vi "ExecuteXML.vi"(0 "reference in":refnum<class "ViPER.lvclass">, 1 "XML_In":string, 3 "get_prototype":bool, 5 "error in (no error)":errorcluster) -> (14 "reference out":refnum<class "ViPER.lvclass">, 15 "XML_Out":string, 19 "error out":errorcluster)   [LabVIEW 2019]
doc: "### BSD License (http://www.opensource.org/licenses/bsd-license.php) Begin ###\n\nCopyright (c) 2018 Kurt Friday www.medulla.net\n\nAll rights reserved.\n\nRedistribution and use in source and binary forms, with or without\nmodification, are permitted provided that the following conditions are met:\n\n * Redistributions of source code must retain the above copyright\n notice, this list of conditions and the following disclaimer.\n\n * Redistributions in binary form must reproduce the above copyright\n notice, this list of conditions and the following disclaimer in the\n documentation and/or other materials provided with the distribution.\n\n * Neither the name of the <organization> nor the\n names of its contributors may be used to endorse or promote products\n derived from this software without specific prior written permission.\n\nTHIS SOFTWARE IS PROVIDED BY THE COPYRIGHT HOLDERS AND CONTRIBUTORS \"AS IS\" AND\nANY EXPRESS OR IMPLIED WARRANTIES, INCLUDING, BUT NOT LIMITED TO, THE IMPLIED\nWARRANTIES OF MERCHANTABILITY AND FITNESS FOR A PARTICULAR PURPOSE ARE\nDISCLAIMED. IN NO EVENT SHALL <COPYRIGHT HOLDER> BE LIABLE FOR ANY\nDIRECT, INDIRECT, INCIDENTAL, SPECIAL, EXEMPLARY, OR CONSEQUENTIAL DAMAGES\n(INCLUDING, BUT NOT LIMITED TO, PROCUREMENT OF SUBSTITUTE GOODS OR SERVICES;\nLOSS OF USE, DATA, OR PROFITS; OR BUSINESS INTERRUPTION) HOWEVER CAUSED AND\nON ANY THEORY OF LIABILITY, WHETHER IN CONTRACT, STRICT LIABILITY, OR TORT\n(INCLUDING NEGLIGENCE OR OTHERWISE) ARISING IN ANY WAY OUT OF THE USE OF THIS\nSOFTWARE, EVEN IF ADVISED OF THE POSSIBILITY OF SUCH DAMAGE."
uses:
  ViPER.lvclass
  <vilib>/xml/NI_XML.lvlib
  <vilib>/xml/Close Reference(Node).vi
  <resource>/objmgr/DOMUserDefRef.rc
  <vilib>/xml/Load XML String.vi
  <userlib>/_OpenG.lib/string/string.llb/Trim Whitespace (String)__ogtk.vi
panel:
  # "### BSD License (http://www.opensource.org/licenses/bsd-license.php) Begin ###\n\nCopyright (c) 2018  Kurt Friday www.medulla.net\n\nAll rights reserved.\n\nRedistribution and use in source and binary forms, with or without\nmodification, are permitted provided that the following conditions are met:\n\n    * Redistributions of source code must retain the above copyright\n      notice, this list of conditions and the following disclaimer.\n\n    * Redistributions in binary form must reproduce the above copyright\n      notice, this list of conditions and the following disclaimer in the\n      documentation and/or other materials provided with the distribution.\n\n    * Neither the name of the <organization> nor the\n      names of its contributors may be used to endorse or promote products\n      derived from this software without specific prior written permission.\n\nTHIS SOFTWARE IS PROVIDED BY THE COPYRIGHT HOLDERS AND CONTRIBUTORS \"AS IS\" AND\nANY EXPRESS OR IMPLIED WARRANTIES, INCLUDING, BUT NOT LIMITED TO, THE IMPLIED\nWARRANTIES OF MERCHANTABILITY AND FITNESS FOR A PARTICULAR PURPOSE ARE\nDISCLAIMED. IN NO EVENT SHALL <COPYRIGHT HOLDER> BE LIABLE FOR ANY\nDIRECT, INDIRECT, INCIDENTAL, SPECIAL, EXEMPLARY, OR CONSEQUENTIAL DAMAGES\n(INCLUDING, BUT NOT LIMITED TO, PROCUREMENT OF SUBSTITUTE GOODS OR SERVICES;\nLOSS OF USE, DATA, OR PROFITS; OR BUSINESS INTERRUPTION) HOWEVER CAUSED AND\nON ANY THEORY OF LIABILITY, WHETHER IN CONTRACT, STRICT LIABILITY, OR TORT\n(INCLUDING NEGLIGENCE OR OTHERWISE) ARISING IN ANY WAY OUT OF THE USE OF THIS\nSOFTWARE, EVEN IF ADVISED OF THE POSSIBILITY OF SUCH DAMAGE."
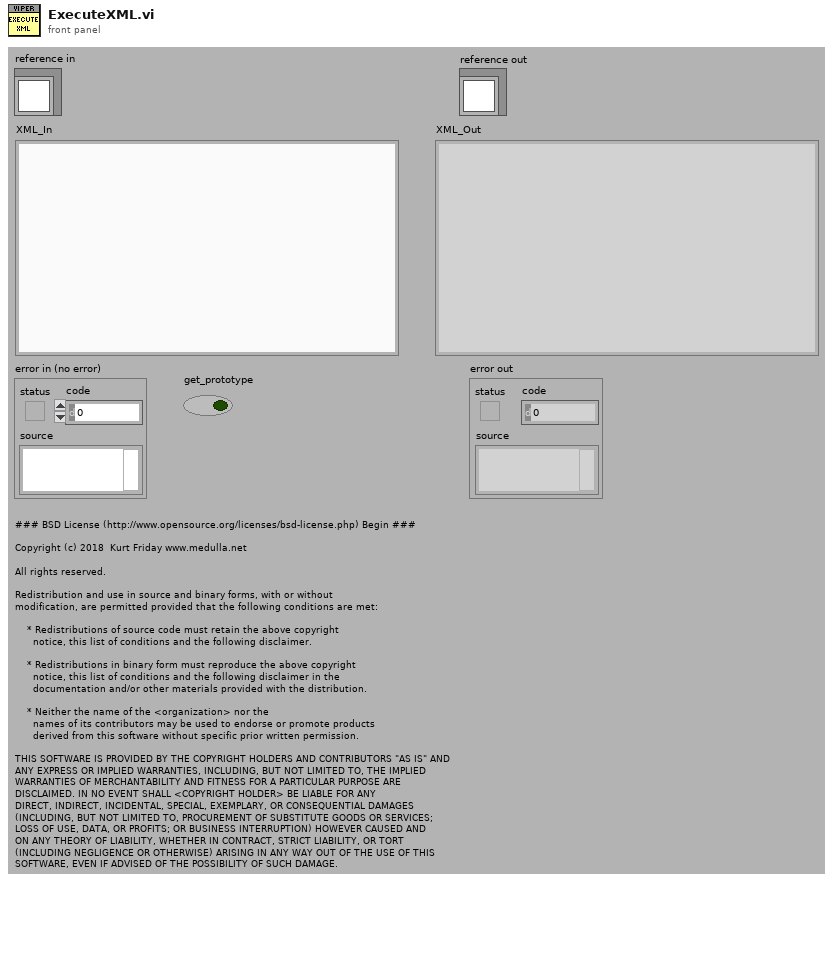
[diagram p1: front panel]
types:
  T1 = cluster{"Method":string, "Wait_Done":bool, "Options":i32, "Inputs":string[]}
  T2 = typedef "ViPER.lvlib/ViPER.lvclass/ObjectAttributes.ctl" = cluster{"Object":T3, "Ancestors":T5[], "Config":T6, "Init_OK":bool, "Hierachy":string[], "PPL?":bool[], "SFP_Open":bool[], "Attributes_SFP_Open":bool[], "Config_SFP_Open":bool[], "SoftFP_event":refnum<user-event>[], "ConfigFP_event":refnum<user-event>[], "AttributesFP_event":refnum<user-event>[], "SoftFP_Shutdown_Notifier":refnum<notifier>[], "ConfigFP_Shutdown_Notifier":refnum<notifier>[], "AttributesFP_Shutdown_Notifier":refnum<notifier>[]}
  T3 = typedef "ViPER.lvlib/ViPER.lvclass/ObjectDefinition.ctl" = cluster{"Name":string, "Ancestors":T4[]}
  T4 = typedef "ViPER.lvlib/ViPER.lvclass/Ancestor.ctl" = cluster{"Class":string, "Config":string, "Objects":string[]}
  T5 = typedef "ViPER.lvlib/ViPER.lvclass/ObjectLayers.ctl" = cluster{"Ancestor":string, "Objects":refnum<class "ViPER.lvclass">[], "Object_Names":string[], "Owned":bool[]}
  T6 = typedef "ViPER.lvlib/ViPER.lvclass/Config.ctl" = cluster{"default":string}
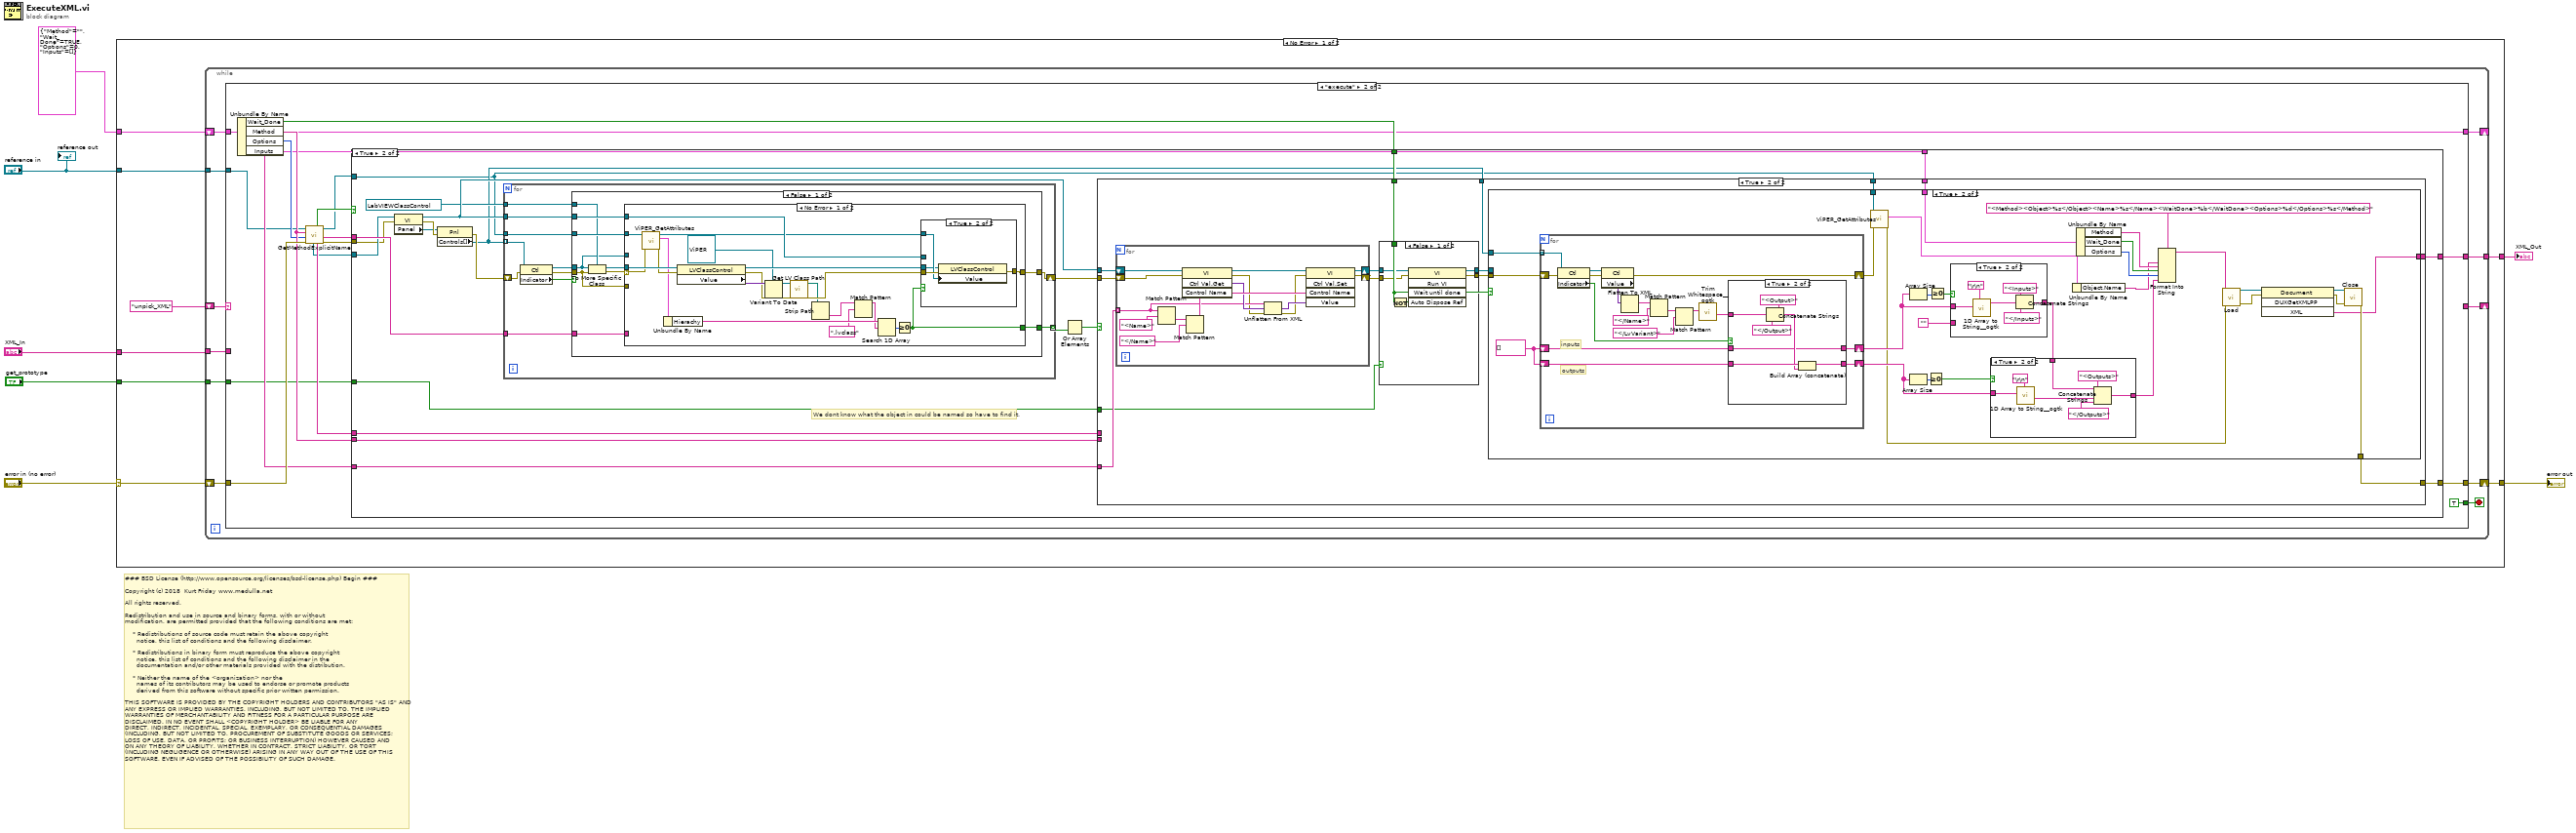
[diagram p0: block diagram]
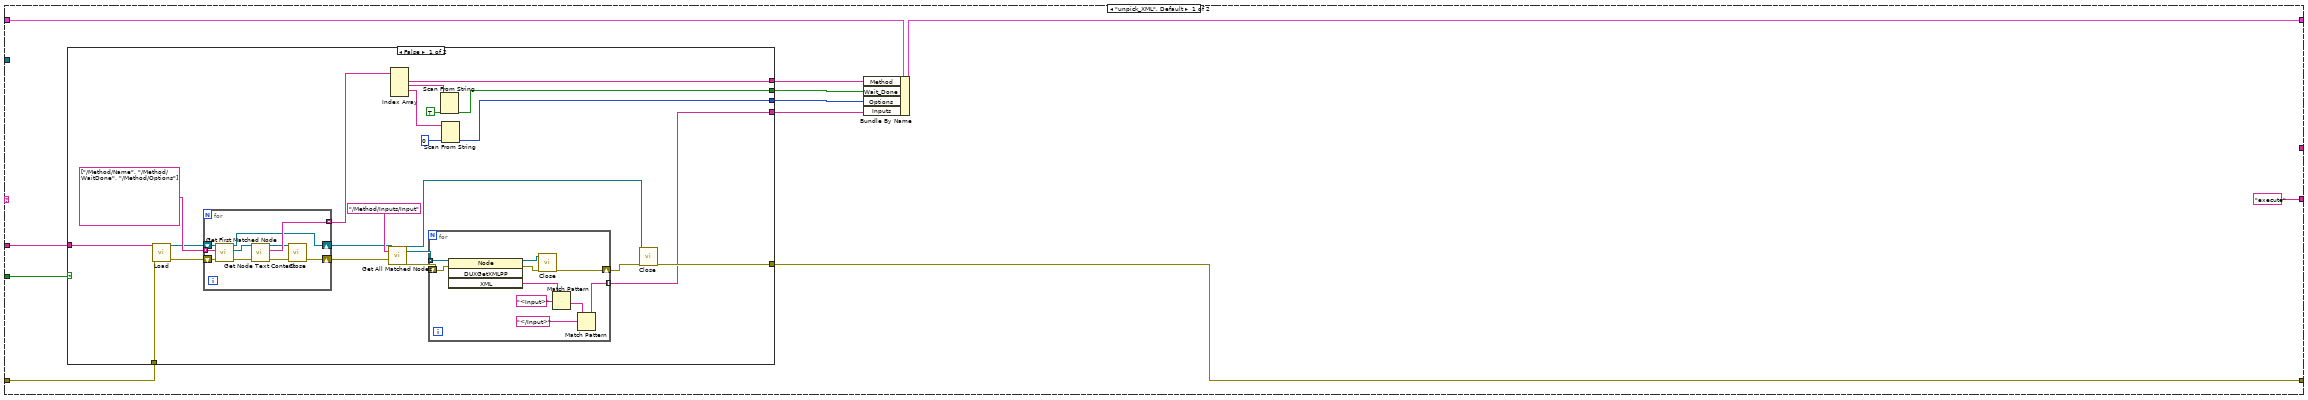
[diagram p2: hidden frame]
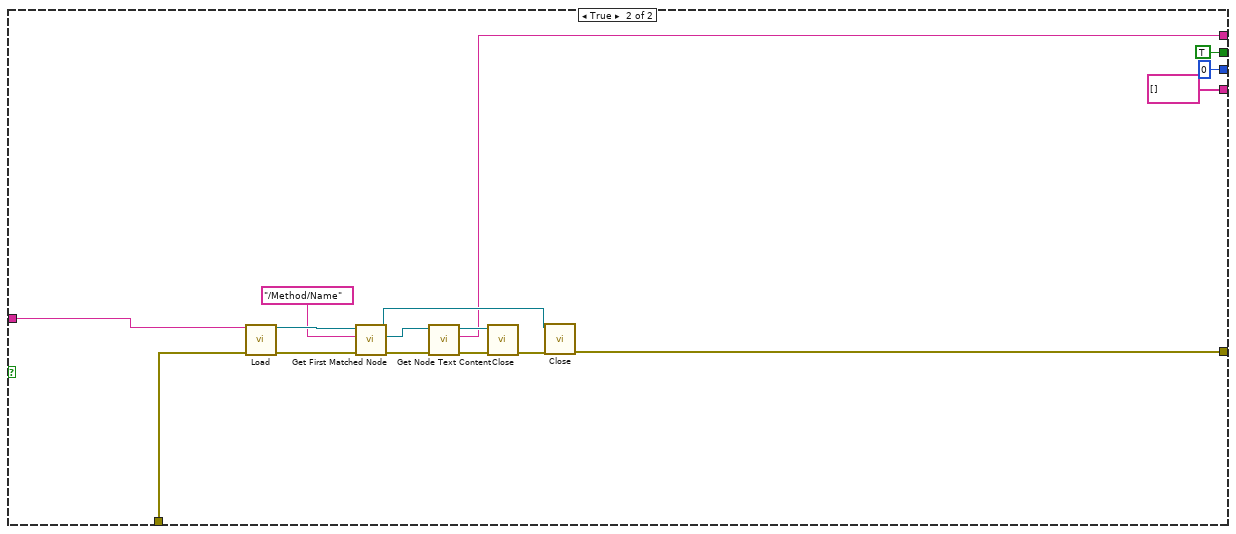
[diagram p3: hidden frame]
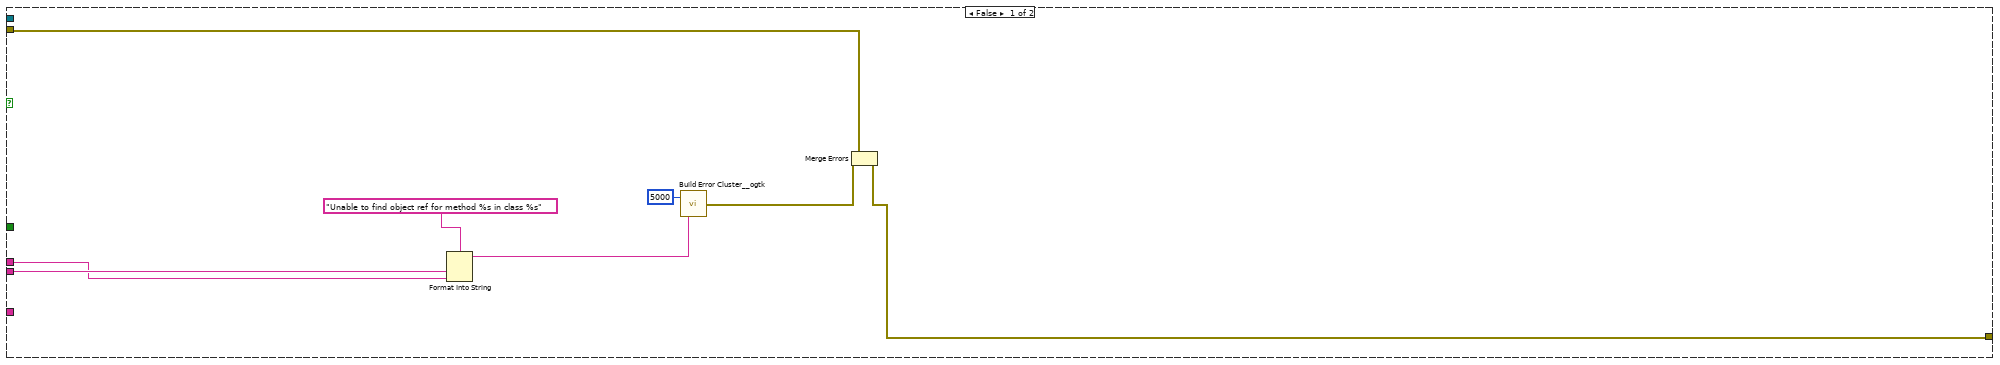
[diagram p5: hidden frame]
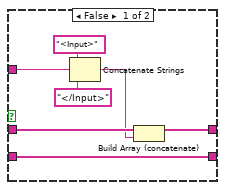
[diagram p10: hidden frame]
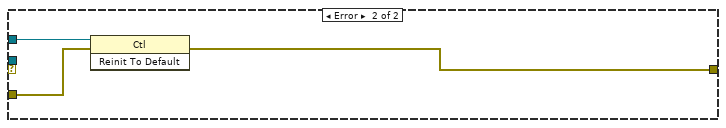
[diagram p12: hidden frame]
diagram:
  # "### BSD License (http://www.opensource.org/licenses/bsd-license.php) Begin ###\n\nCopyright (c) 2018  Kurt Friday www.medulla.net\n\nAll rights reserved.\n\nRedistribution and use in source and binary forms, with or without\nmodification, are permitted provided that the following conditions are met:\n\n    * Redistributions of source code must retain the above copyright\n      notice, this list of conditions and the following disclaimer.\n\n    * Redistributions in binary form must reproduce the above copyright\n      notice, this list of conditions and the following disclaimer in the\n      documentation and/or other materials provided with the distribution.\n\n    * Neither the name of the <organization> nor the\n      names of its contributors may be used to endorse or promote products\n      derived from this software without specific prior written permission.\n\nTHIS SOFTWARE IS PROVIDED BY THE COPYRIGHT HOLDERS AND CONTRIBUTORS \"AS IS\" AND\nANY EXPRESS OR IMPLIED WARRANTIES, INCLUDING, BUT NOT LIMITED TO, THE IMPLIED\nWARRANTIES OF MERCHANTABILITY AND FITNESS FOR A PARTICULAR PURPOSE ARE\nDISCLAIMED. IN NO EVENT SHALL <COPYRIGHT HOLDER> BE LIABLE FOR ANY\nDIRECT, INDIRECT, INCIDENTAL, SPECIAL, EXEMPLARY, OR CONSEQUENTIAL DAMAGES\n(INCLUDING, BUT NOT LIMITED TO, PROCUREMENT OF SUBSTITUTE GOODS OR SERVICES;\nLOSS OF USE, DATA, OR PROFITS; OR BUSINESS INTERRUPTION) HOWEVER CAUSED AND\nON ANY THEORY OF LIABILITY, WHETHER IN CONTRACT, STRICT LIABILITY, OR TORT\n(INCLUDING NEGLIGENCE OR OTHERWISE) ARISING IN ANY WAY OUT OF THE USE OF THIS\nSOFTWARE, EVEN IF ADVISED OF THE POSSIBILITY OF SUCH DAMAGE."
  n1 = case shown="No Error" "error in (no error)" {
    selector: "error in (no error)" -> [w14 w307]
    tunnel: [w15 w307] -> w6
    tunnel: "reference in" -> [w9 _]
    tunnel: "XML_In" -> [w13 _]
    tunnel: T1 {"Method"="", "Wait_Done"=TRUE, "Options"=0, "Inputs"=[]} -> [w11 _]
    tunnel: [w10 _] -> w3
    tunnel: "get_prototype" -> [w8 _]
    frame No Error {
      n2 = while {
        shift-right: [w26] -> w15
        shift-left: w14 -> [w25]
        tunnel: w13 -> [w24]
        shift-right: [w19] -> _
        shift-left: "unpick_XML" -> [w23]
        shift-right: [w21] -> _
        shift-left: w11 -> [w22]
        tunnel: [w18] -> w10
        tunnel: w9 -> [w17]
        tunnel: w8 -> [w16]
        stop <- w20 stop-if-true
        n3 = case shown="\"execute\"" w23 {
          tunnel: [w28 w112] -> w26
          tunnel: w25 -> [w36 w109]
          tunnel: w24 -> [w37 _]
          tunnel: w22 -> [w35 w100]
          tunnel: [w30 w100] -> w21
          tunnel: [_ TRUE] -> w20
          tunnel: ["execute" _] -> w19
          tunnel: [_ w99] -> w18
          tunnel: w17 -> [_ w97]
          tunnel: w16 -> [w27 w96]
          frame "unpick_XML", Default {
            n4 = case shown="False" w27 {
              tunnel: w37 -> [w51 w95]
              tunnel: w36 -> [w50 w94]
              tunnel: [w46 w83] -> w34
              tunnel: [w43 TRUE] -> w33
              tunnel: [w40 0 ("options")] -> w32
              tunnel: [w38 string[] []] -> w31
              tunnel: [w39 w84] -> w28
              frame False {
                n5 = call-poly <vilib>:"Load.vi"("XML string"=w51, "error in (no error)"=w50) -> ("DOM document out"=w52:refnum<k20>, "error out"=w53:errorcluster)  [unwired: 11 in, 1 out]
                n6 = for {
                  tunnel: string[] ["/Method/Name", "/Method/WaitDone", "/Method/Options"] -> [w75] mode=indexing
                  tunnel: [w74] -> w47 mode=indexing
                  shift-right: [w71] -> w55
                  shift-left: w53 -> [w78]
                  shift-right: [w70] -> w56
                  shift-left: w52 -> [w79]
                  n7 = call <vilib>:"Get First Matched Node.vi"("error in (no error)"=w78, "XPath expression"=w75, "node in"=w79) -> ("error out"=w76:errorcluster, "node result"=w77:refnum<k20>, "node out"=w70:refnum<k20>)  [unwired: 6 in]
                  n8 = call <vilib>:"Get Node Text Content.vi"("error in (no error)"=w76, "node in"=w77) -> ("error out"=w73:errorcluster, "node text"=w74:string, "node out"=w72:refnum<k20>)  [unwired: 7 in]
                  n9 = call-poly <vilib>:"Close.vi"("error in (no error)"=w73, "node"=w72) -> ("error out"=w71:errorcluster)  [unwired: 7 in]
                }
                n10 = call <vilib>:"Get All Matched Nodes.vi"("error in (no error)"=w55, "XPath expression"="/Method/Inputs/Input", "node in"=w56) -> ("error out"=w59:errorcluster, "node result array"=w58:refnum<k20>[], "node out"=w48:refnum<k20>)  [unwired: 6 in]
                n11 = Index Array(array=w47) -> (element #1=w46:string, element #2=w45:string, element #3=w42:string)  [unwired: 4 in, 1 out]
                n12 = for {
                  tunnel: w58 -> [w69] mode=indexing
                  shift-right: [w66] -> w49
                  shift-left: w59 -> [w68]
                  tunnel: [w60] -> w38 mode=indexing
                  n13 = invoke class="Node" method="DUXGetXMLPP"(reference=w69, error in=w68) -> (reference out=w65:refnum<k20>, error out=w67:errorcluster, "XML"=w61:string)  [unwired: 2 in, 1 out]
                  n14 = call-poly <vilib>:"Close.vi"("error in (no error)"=w67, "node"=w65) -> ("error out"=w66:errorcluster)  [unwired: 7 in]
                  n15 = Match Pattern(string=w61, regular expression="<Input>") -> (after substring=w63:string)  [unwired: 1 in, 3 out]
                  n16 = Match Pattern(string=w63, regular expression="</Input>") -> (before substring=w60:string)  [unwired: 1 in, 3 out]
                }
                n17 = Scan From String(input string=w45, default 1=TRUE) -> (output 1=w43:bool)  [unwired: 3 in, 3 out]
                n18 = Scan From String(input string=w42, default 1=0 ("options")) -> (output 1=w40:i32)  [unwired: 3 in, 3 out]
                n19 = call-poly <vilib>:"Close.vi"("error in (no error)"=w49, "node"=w48) -> ("error out"=w39:errorcluster)  [unwired: 7 in]
              }
              frame True {
                n20 = call-poly <vilib>:"Load.vi"("XML string"=w95, "error in (no error)"=w94) -> ("DOM document out"=w92:refnum<k20>, "error out"=w93:errorcluster)  [unwired: 11 in, 1 out]
                n21 = call <vilib>:"Get First Matched Node.vi"("error in (no error)"=w93, "XPath expression"="/Method/Name", "node in"=w92) -> ("error out"=w90:errorcluster, "node result"=w89:refnum<k20>, "node out"=w85:refnum<k20>)  [unwired: 6 in]
                n22 = call <vilib>:"Get Node Text Content.vi"("error in (no error)"=w90, "node in"=w89) -> ("error out"=w87:errorcluster, "node text"=w83:string, "node out"=w88:refnum<k20>)  [unwired: 7 in]
                n23 = call-poly <vilib>:"Close.vi"("error in (no error)"=w87, "node"=w88) -> ("error out"=w86:errorcluster)  [unwired: 7 in]
                n24 = call-poly <vilib>:"Close.vi"("error in (no error)"=w86, "node"=w85) -> ("error out"=w84:errorcluster)  [unwired: 7 in]
              }
            }
            n25 = Bundle By Name(cluster=w35, "Method"=w34, "Wait_Done"=w33, "Options"=w32, "Inputs"=w31) -> (w30:T1)
          }
          frame "execute" {
            n26 = Unbundle By Name(w100) -> ("Wait_Done"=w103:bool, "Method"=w105:string, "Options"=w104:i32, "Inputs"=w102:string[])
            n27 = call "GetMethodExplicitName.vi"("error in (no error)"=w109, "options"=w104, "method"=w105, "Driver in"=w97) -> ("error out"=w107:errorcluster, "class explicit name"=w111:string, "Driver out"=w98:refnum<class "ViPER.lvclass">, "class"=w110:string, "exists"=w106:bool, "vi reference"=w108:refnum<vi>)  [unwired: 1 in, 1 out]
            n28 = case shown="True" w106 {
              tunnel: [w113 w134] -> w112
              tunnel: w111 -> [_ w128]
              tunnel: w110 -> [_ w127]
              tunnel: w105 -> [_ w126]
              tunnel: w98 -> [_ w114]
              tunnel: w108 -> [_ w122]
              tunnel: w107 -> [w113 w121]
              tunnel: w103 -> [_ w120]
              tunnel: w102 -> [_ w119]
              tunnel: w100 -> [_ w117]
              tunnel: [_ w116] -> w99
              tunnel: w96 -> [_ w115]
              frame False {
              }
              frame True {
                # "We dont know what the object in could be named so have to find it."
                n29 = property class="VI"(reference=w122, error in=w121) -> (reference out=w132:refnum<vi>, error out=w133:errorcluster, "Panel"=w125:refnum<vi>)
                n30 = property class="Pnl"(reference=w125, error in=w133) -> (error out=w131:errorcluster, "Controls[]"=w118:refnum<vi>[])  [unwired: 1 out]
                n31 = for {
                  tunnel: w118 -> [w255] mode=indexing
                  tunnel: w128 -> [w262]
                  tunnel: w114 -> [w260]
                  tunnel: w132 -> [w261]
                  shift-right: [w259] -> w130
                  shift-left: w131 -> [w256]
                  tunnel: [w258] -> w124 mode=indexing
                  tunnel: refnum<vi> refnum ("reference in") -> [w257]
                  n32 = property class="Ctl"(reference=w255, error in=w256) -> (reference out=w265:refnum<vi>, error out=w264:errorcluster, "Indicator"=w263:bool)
                  n33 = case shown="False" w263 {
                    tunnel: w265 -> [w266 _]
                    tunnel: w264 -> [w267 w306]
                    tunnel: w262 -> [w273 _]
                    tunnel: [w272 _] -> w258
                    tunnel: w261 -> [w271 _]
                    tunnel: w260 -> [w270 _]
                    tunnel: [w269 w306] -> w259
                    tunnel: w257 -> [w268 _]
                    frame False {
                      n34 = To More Specific Class(target class=w268, reference=w266, error in=w267) -> (specific class reference=w275:refnum<vi>, error out=w274:errorcluster)
                      n35 = case shown="No Error" w274 {
                        selector: w274 -> [w284 _]
                        tunnel: w275 -> [w288 _]
                        tunnel: w273 -> [_ _]
                        tunnel: [w276 _] -> w272
                        tunnel: w271 -> [w296 _]
                        tunnel: w270 -> [w286 _]
                        tunnel: w267 -> [_ w304]
                        tunnel: [w295 w303] -> w269
                        tunnel: w266 -> [_ w305]
                        frame No Error {
                          n36 = call "ViPER_GetAttributes.vi"("error in (no error)"=w284, "reference in"=w286) -> ("error out"=w283:errorcluster, "Data"=w282:T2, "reference out"=w285:refnum<class "ViPER.lvclass">)  [unwired: 6 in, 1 out]
                          n37 = Unbundle By Name(w282) -> ("Hierachy"=w281:string[])
                          n38 = property class="LVClassControl"(reference=w288, error in=w283) -> (reference out=w297:refnum<vi>, error out=w291:errorcluster, "Value"=w292:variant)
                          n39 = Variant To Data(error in=w291, type=refnum<class "ViPER.lvclass"> refnum ("Driver in"), Variant=w292) -> (data=w289:refnum<class "ViPER.lvclass">, error out=w290:errorcluster)
                          n40 = call <vilib>:"Get LV Class Path.vi"("error in (no error)"=w290, "object"=w289) -> ("error out"=w294:errorcluster, "class path"=w293:path)  [unwired: 8 in]
                          n41 = Strip Path(path=w293) -> (name=w279:string)  [unwired: 1 out]
                          n42 = Match Pattern(string=w279, regular expression=".lvclass") -> (before substring=w278:string)  [unwired: 1 in, 3 out]
                          n43 = Search 1D Array(1D array=w281, element=w278) -> (index of element=w277:i32)  [unwired: 1 in]
                          n44 = Greater Or Equal To 0?(x=w277) -> (x >= 0?=w276:bool)
                          n45 = case shown="True" w276 {
                            tunnel: w297 -> [_ w299]
                            tunnel: w294 -> [w298 w302]
                            tunnel: w296 -> [_ _]
                            tunnel: w285 -> [_ w301]
                            tunnel: [w298 w300] -> w295
                            frame False {
                            }
                            frame True {
                              n46 = property class="LVClassControl"(reference=w299, error in=w302, "Value"=w301) -> (error out=w300:errorcluster)  [unwired: 1 out]
                            }
                          }
                        }
                        frame Error {
                          n47 = invoke class="Ctl" method="Reinit To Default"(reference=w305, error in=w304) -> (error out=w303:errorcluster)  [unwired: 1 in, 2 out]
                        }
                      }
                    }
                    frame True {
                    }
                  }
                }
                n48 = Or Array Elements(Boolean array=w124) -> (logical OR=w123:bool)
                n49 = case shown="True" w123 {
                  tunnel: [w136 w145] -> w134
                  tunnel: w132 -> [_ w152]
                  tunnel: w130 -> [w135 w151]
                  tunnel: w126 -> [w141 _]
                  tunnel: w127 -> [w140 _]
                  tunnel: w120 -> [_ w150]
                  tunnel: w119 -> [_ w149]
                  tunnel: w118 -> [_ w148]
                  tunnel: w117 -> [_ w147]
                  tunnel: [_ w146] -> w116
                  tunnel: w115 -> [_ w144]
                  tunnel: w114 -> [_ w143]
                  frame False {
                    n50 = Format Into String(format string="Unable to find object ref for method %s in class %s", w141, w140) -> (resulting string=w138:string)  [unwired: 2 in, 1 out]
                    n51 = call <userlib>:"Build Error Cluster__ogtk.vi"("String to Prepend to source (\"\")"=w138, "code"=5000) -> ("error out"=w137:errorcluster)
                    n52 = Merge Errors(w135, w137) -> (w136:errorcluster)
                  }
                  frame True {
                    n53 = for {
                      shift-right: [w253] -> w155
                      shift-left: w151 -> [w247]
                      shift-right: [w254] -> w156
                      shift-left: w152 -> [w249]
                      tunnel: w149 -> [w244] mode=indexing
                      n54 = Match Pattern(string=w244, regular expression="<Name>") -> (after substring=w251:string)  [unwired: 1 in, 3 out]
                      n55 = Match Pattern(string=w251, regular expression="</Name>") -> (before substring=w246:string)  [unwired: 1 in, 3 out]
                      n56 = invoke class="VI" method="Ctrl Val.Get"(reference=w249, error in=w247, "Control Name"=w246) -> (reference out=w248:refnum<vi>, error out=w242:errorcluster, "Get Control Value Variant"=w245:variant)  [unwired: 1 in, 1 out]
                      n57 = Unflatten From XML(xml string=w244, type=w245, error in (no error)=w242) -> (value=w243:variant, error out=w241:errorcluster)
                      n58 = invoke class="VI" method="Ctrl Val.Set"(reference=w248, error in=w241, "Control Name"=w246, "Value"=w243) -> (reference out=w254:refnum<vi>, error out=w253:errorcluster)  [unwired: 1 in, 3 out]
                    }
                    n59 = case shown="False" w144 {
                      tunnel: w156 -> [w162 w163]
                      tunnel: w155 -> [w161 w164]
                      tunnel: [w160 w163] -> w154
                      tunnel: [w159 w164] -> w153
                      tunnel: w150 -> [w157 _]
                      frame False {
                        n60 = Not(x=w157) -> (.not. x?=w158:bool)
                        n61 = invoke class="VI" method="Run VI"(reference=w162, error in=w161, "Wait until done"=w157, "Auto Dispose Ref"=w158) -> (reference out=w160:refnum<vi>, error out=w159:errorcluster)  [unwired: 1 in, 3 out]
                      }
                      frame True {
                      }
                    }
                    n62 = case shown="True" w150 {
                      tunnel: w154 -> [_ _]
                      tunnel: w153 -> [w165 w193]
                      tunnel: w148 -> [_ w194]
                      tunnel: w147 -> [_ w184]
                      tunnel: [_ w172] -> w146
                      tunnel: [w165 w174] -> w145
                      tunnel: w143 -> [_ w168]
                      frame False {
                      }
                      frame True {
                        w192 = string[] []
                        n63 = for {
                          tunnel: w194 -> [w218] mode=indexing
                          shift-right: [w223] -> w170
                          shift-left: w193 -> [w226]
                          shift-right: [w219] -> w189
                          shift-left: w192 -> [w221]
                          shift-right: [w220] -> w188
                          shift-left: w192 -> [w222]
                          # "outputs"
                          # "inputs"
                          n64 = property class="Ctl"(reference=w218, error in=w226) -> (reference out=w225:refnum<vi>, error out=w224:errorcluster, "Indicator"=w217:bool)
                          n65 = property class="Ctl"(reference=w225, error in=w224) -> (error out=w223:errorcluster, "Value"=w216:variant)  [unwired: 1 out]
                          n66 = Flatten To XML(anything=w216) -> (xml string=w215:string)
                          n67 = Match Pattern(string=w215, regular expression="</Name>") -> (after substring=w213:string)  [unwired: 1 in, 3 out]
                          n68 = Match Pattern(string=w213, regular expression="</LvVariant>") -> (before substring=w211:string)  [unwired: 1 in, 3 out]
                          n69 = call-poly <userlib>:"Trim Whitespace__ogtk.vi"("String in"=w211) -> ("String out"=w210:string)  [unwired: 6 in]
                          n70 = case shown="True" w217 {
                            tunnel: w210 -> [w230 w240]
                            tunnel: w221 -> [w229 w234]
                            tunnel: w222 -> [w233 w236]
                            tunnel: [w233 w237] -> w220
                            tunnel: [w227 w234] -> w219
                            frame False {
                              n71 = Concatenate Strings("<Input>" ("string"), w230, "</Input>" ("string")) -> (w228:string)
                              n72 = Build Array (concatenate)(w229, w228) -> (w227:string[])
                            }
                            frame True {
                              n73 = Concatenate Strings("<Output>" ("string"), w240, "</Output>" ("string")) -> (w235:string)
                              n74 = Build Array (concatenate)(w236, w235) -> (w237:string[])
                            }
                          }
                        }
                        n75 = call "ViPER_GetAttributes.vi"("error in (no error)"=w170, "reference in"=w168) -> ("error out"=w169:errorcluster, "Data"=w167:T2)  [unwired: 6 in, 2 out]
                        n76 = Array Size(array=w189) -> (size(s)=w191:i32)
                        n77 = Array Size(array=w188) -> (size(s)=w190:i32)
                        n78 = Greater Or Equal To 0?(x=w190) -> (x >= 0?=w179:bool)
                        n79 = Greater Or Equal To 0?(x=w191) -> (x >= 0?=w180:bool)
                        n80 = case shown="True" w180 {
                          tunnel: w189 -> [_ w209]
                          tunnel: [w203 w204] -> w186
                          tunnel: "" -> [w203 _]
                          frame False {
                          }
                          frame True {
                            n81 = call <userlib>:"1D Array to String__ogtk.vi"("delimiter (Tab)"="\r\n", "Array of Strings"=w209) -> ("delimited string"=w205:string)  [unwired: 9 in]
                            n82 = Concatenate Strings("<Inputs>" ("string"), w205, "</Inputs>" ("string")) -> (w204:string)
                          }
                        }
                        n83 = case shown="True" w179 {
                          tunnel: w188 -> [_ w202]
                          tunnel: [w195 w197] -> w171
                          tunnel: w186 -> [w195 w196]
                          frame False {
                          }
                          frame True {
                            n84 = call <userlib>:"1D Array to String__ogtk.vi"("delimiter (Tab)"="\r\n", "Array of Strings"=w202) -> ("delimited string"=w198:string)  [unwired: 9 in]
                            n85 = Concatenate Strings(w196, "<Outputs>" ("string"), w198, "</Outputs>" ("string")) -> (w197:string)
                          }
                        }
                        n86 = Unbundle By Name(w167) -> ("Object.Name"=w166:string)
                        n87 = Unbundle By Name(w184) -> ("Method"=w183:string, "Wait_Done"=w182:bool, "Options"=w181:i32)
                        n88 = Format Into String(format string="<Method><Object>%s</Object><Name>%s</Name><WaitDone>%b</WaitDone><Options>%d</Options>%s</Method>", w166, w183, w182, w181, w171) -> (resulting string=w173:string)  [unwired: 2 in, 1 out]
                        n89 = call-poly <vilib>:"Load.vi"("XML string"=w173, "error in (no error)"=w169) -> ("DOM document out"=w178:refnum<k20>, "error out"=w177:errorcluster)  [unwired: 11 in, 1 out]
                        n90 = invoke class="Document" method="DUXGetXMLPP"(reference=w178, error in=w177) -> (reference out=w176:refnum<k20>, error out=w175:errorcluster, "XML"=w172:string)  [unwired: 2 in, 1 out]
                        n91 = call-poly <vilib>:"Close.vi"("error in (no error)"=w175, "node"=w176) -> ("error out"=w174:errorcluster)  [unwired: 7 in]
                      }
                    }
                  }
                }
              }
            }
          }
        }
      }
    }
    frame Error {
    }
  }
  "error out" <- w6
  "XML_Out" <- w3
  "reference out" <- "reference in"
